vi "Create.vi"(8 "error in (no error)":errorcluster, 9 "Path":path, 10 "ID":string, 11 "class1 in":refnum<class "class1.lvclass">) -> (0 "error out":errorcluster, 3 "class1 out":refnum<class "class1.lvclass">)   [LabVIEW 2018, in "class1.lvclass"]
uses:
  class1.lvclass
  class1.lvclass/class1.ctl
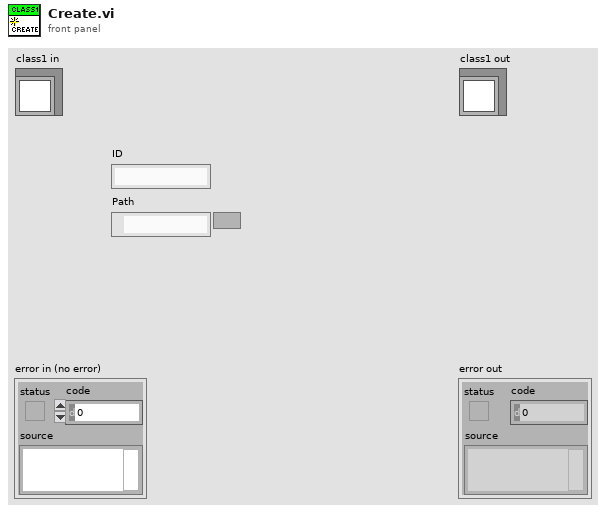
[diagram p1: front panel]
types:
  T1 = typedef "class1.lvclass/Data.ctl" = cluster{"Path":path, "ID":string, "Settings":T2, "asdf":enum16{"a", "f"}, "XY Graph":cluster{"X":dbl, "Y":dbl}[]}
  T2 = typedef "class1.lvclass/Settings.ctl" = cluster{"Speed":dbl, "Strr":string, "data":i32[]}
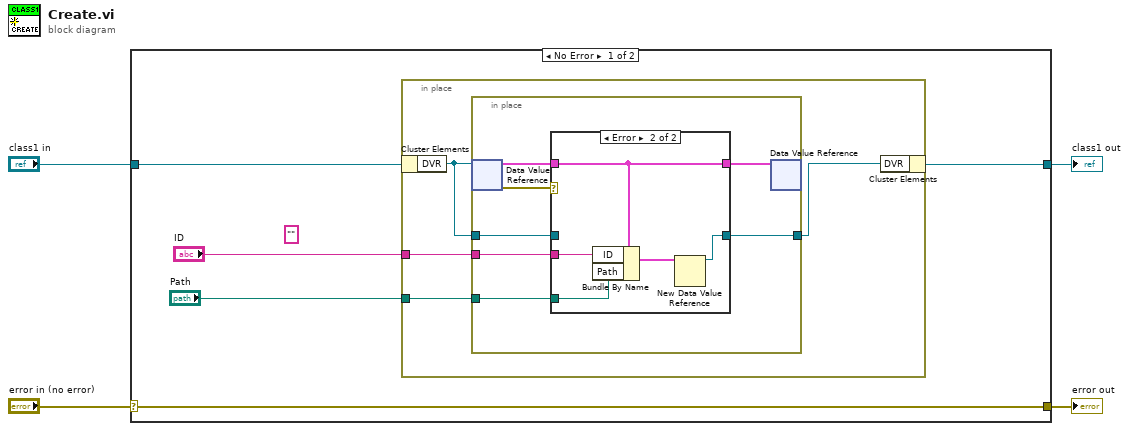
[diagram p0: block diagram]
diagram:
  n1 = case shown="No Error" "error in (no error)" {
    selector: "error in (no error)" -> [w5 w29]
    tunnel: [w5 w29] -> w3
    tunnel: [w6 w28] -> w1
    tunnel: "class1 in" -> [w9 w28]
    frame No Error {
      (unwired) ""
      n2 = in-place {
        in-place-border: "ID" -> [w13]
        in-place-border: "Path" -> [w12]
        n3 = in-place-cluster #1(w9) -> ("DVR"=w11:refnum<data-value>)
        n4 = in-place {
          in-place-border: w13 -> [w19]
          in-place-border: w12 -> [w18]
          in-place-border: [w15] -> w10
          in-place-border: w11 -> [w14]
          n5 = in-place-dvr #2(w11) -> (w17:T1, w20:errorcluster)
          n6 = case shown="Error" w20 {
            tunnel: w19 -> [_ w27]
            tunnel: w18 -> [_ w26]
            tunnel: w17 -> [w22 w23]
            tunnel: [w22 w23] -> w16
            tunnel: [w21 w24] -> w15
            tunnel: w14 -> [w21 _]
            frame No Error {
            }
            frame Error {
              n7 = Bundle By Name(cluster=w23, "ID"=w27, "Path"=w26) -> (w25:T1)
              n8 = New Data Value Reference(data value=w25) -> (data value reference=w24:refnum<data-value>)  [unwired: 1 in, 1 out]
            }
          }
          n9 = in-place-dvr #2(w16) -> ()  [unwired: 2 out]
        }
        n10 = in-place-cluster #1("DVR"=w10) -> (w6:refnum<class "class1.lvclass">)
      }
    }
    frame Error {
    }
  }
  "error out" <- w3
  "class1 out" <- w1
